vi "Send Pre-Addressed Publish.vi"(6 "Publish Time (Use Current Time)":timestamp, 8 "error in (no error)":errorcluster, 9 "Data to Publish":variant, 10 "Topic Name":string, 11 "Publish Message":refnum<class "Publish Msg.lvclass">) -> (0 "error out":errorcluster)   [LabVIEW 2015, in "IMediator.lvlib" / "Publish Msg.lvclass"]
doc: "Most Actors or VIs that want to publish data will do so with this send VI. Actors who call this method must have been given a pre-addressed Publish Msg prior to the act of sending. (For Actors, this means that they were launched with a pre-addressed Publish Msg or sent one after the Mediator came alive.)\n\n<License>\nCopyright © 2017 Composed Systems, LLC | All rights reserved\nwww.composed.io\n\nAuthor: Ethan Stern <ethan.stern@composed.io>\n\nThis software is provided \"AS IS\" WITHOUT WARRANTIES, either express or implied, AND IS FOR EDUCATIONAL PURPOSES ONLY.\n</License>"
uses:
  Publish Msg.lvclass
  AbstractMessages/PreAddressedMsg/PreAddressedMsg.lvclass/PreAddressedMsg.ctl
  Publish Msg.lvclass/Publish Msg.ctl
  <vilib>/ActorFramework/Message Enqueuer/Message Enqueuer.lvclass/Message Enqueuer.ctl
  <vilib>/ActorFramework/Message Priority Queue/Priority Enqueue.vi
  <vilib>/ActorFramework/Message Enqueuer/Message Enqueuer.lvclass
  AbstractMessages/PreAddressedMsg/PreAddressedMsg.lvclass
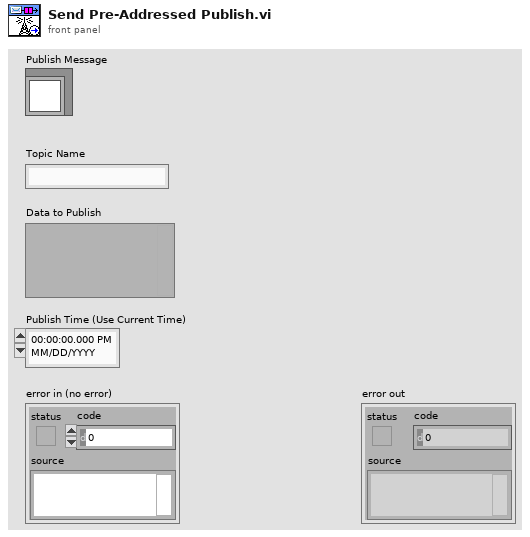
[diagram p1: front panel]
types:
  T1 = typedef "Actor Framework.lvlib/Message Enqueuer.lvclass/Message Priority.ctl" = enum16{"Low", "Normal", "High"}
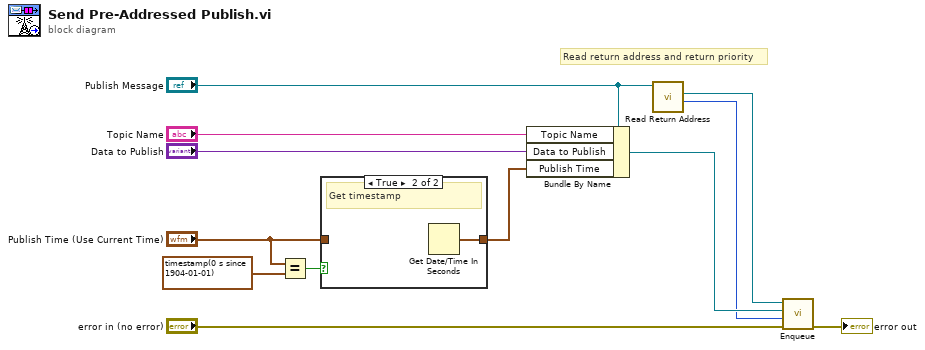
[diagram p0: block diagram]
diagram:
  # "Read return address and return priority"
  n1 = Equal?(x="Publish Time (Use Current Time)", y=timestamp(0 s since 1904-01-01)) -> (x = y?=w3:bool)
  n2 = case shown="True" w3 {
    tunnel: "Publish Time (Use Current Time)" -> [w13 _]
    tunnel: [w13 w14] -> w5
    frame False {
      # "Use input time"
    }
    frame True {
      # "Get timestamp"
      n3 = Get Date/Time In Seconds() -> (seconds since 1Jan1904=w14:timestamp)
    }
  }
  n4 = Bundle By Name(cluster="Publish Message", "Topic Name"="Topic Name", "Data to Publish"="Data to Publish", "Publish Time"=w5) -> (w8:refnum<class "Publish Msg.lvclass">)
  n5 = call "Read Return Address.vi"("PreAddressedMsg in"="Publish Message") -> ("Return Priority (Normal)"=w1:T1, "Return Address"=w6:refnum<class "Message Enqueuer.lvclass">)  [unwired: 9 in]
  n6 = call <vilib>:"Enqueue.vi"("error in (no error)"="error in (no error)", "Message Priority (Normal)"=w1, "Message"=w8, "Message Enqueuer in"=w6) -> ("error out"=→"error out":errorcluster)  [unwired: 6 in, 1 out]
